vi "Call Call Back.vi"(6 "Variant":variant, 7 "old values":string[][](array[string]), 8 "error in (no error)":errorcluster, 9 "object ref in":T2, 10 "Table Change":T1, 11 "Column in":refnum<class "Column.lvclass">) -> (0 "error out":errorcluster, 3 "Column Out":refnum<class "Column.lvclass">)   [LabVIEW 2013, in "Table Manager.lvlib" / "Column.lvclass"]
uses:
  Column.lvclass
  TagSelectModule/Source/editor node/object ref.ctl
  <vilib>/NI/Tag Bus Data Framework/Configuration Editor/Classes/Engine Parent/Engine Parent Editor Node.lvclass
  <vilib>/NI/Tag Bus Data Framework/Configuration Editor/Classes/Module editor node/module editor node.lvclass
  Table Manager/Cell Change.ctl
  Column.lvclass/Column.ctl
  Read Call Back VI.vi
  TagSelectModule/Source/editor node/tag select module editor node.lvclass
  Table Manager.lvlib
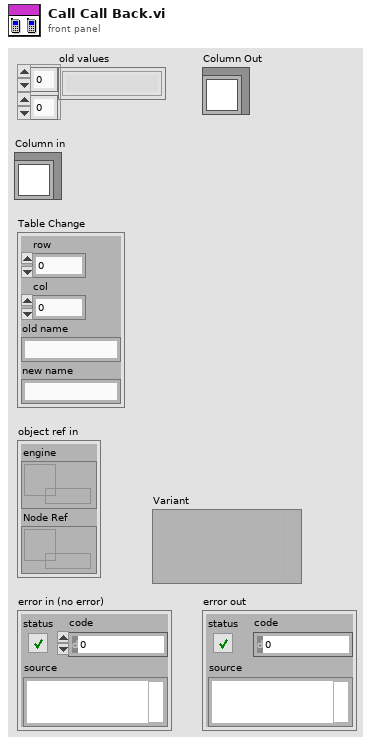
[diagram p1: front panel]
types:
  T1 = typedef "Table Manager.lvlib/Cell Change.ctl" = cluster{"row":i32, "col":i32, "old name":string, "new name":string}
  T2 = typedef "tag select module editor node.lvclass/object ref.ctl" = cluster{"engine":refnum<data-value>, "Node Ref":refnum<data-value>}
  T3 = typedef "Table Manager.lvlib/Column.lvclass/Call Back Ref Type Def.ctl" = refnum<vi>
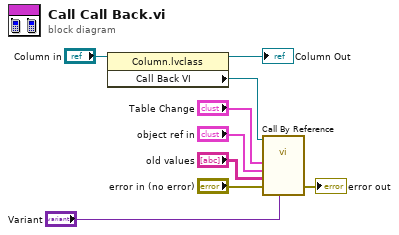
[diagram p0: block diagram]
diagram:
  n1 = property class="Column.lvclass"(reference="Column in") -> (reference out=→"Column Out":refnum<class "Column.lvclass">, "Call Back VI"=w9:T3)  [unwired: 1 in, 1 out]
  n2 = call-by-ref "?"(reference=w9, "Variant"="Variant", "error in (no error)"="error in (no error)", "old values"="old values", "object ref in"="object ref in", "Cluster"="Table Change") -> ("error out"=→"error out":errorcluster)  [unwired: 7 in, 2 out]
